vi "Create Channels From FrontPanel.vi"(8 "error in (no error)":errorcluster, 11 "Controls[]":refnum<vi>[](array[refnum])) -> (0 "error out":errorcluster, 3 "Array":refnum<class "FPGA Channel.lvclass">[](array[class]))   [LabVIEW 2014, in "FPGA Module editor node.lvclass"]
uses:
  FPGA Module editor node.lvclass
  fpga channel/FPGA Channel.lvclass
  <vilib>/NI/Tag Bus Module Framework/channel/channel classification.ctl
  <vilib>/Utility/VariantDataType/Type.ctl
  <vilib>/NI/Tag Bus/tag/Data Type.ctl
  <vilib>/NI/Tag Bus/tag/tag descriptor.lvclass/tag descriptor.ctl
  fpga channel/FPGA Channel.lvclass/FPGA Channel.ctl
  <vilib>/NI/Tag Bus Module Framework/channel/TBM channel.lvclass/TBM channel.ctl
  <vilib>/NI/Tag Bus/tag/write tag name.vi
  <vilib>/NI/Tag Bus/tag/write data type.vi
  fpga channel/Write FXP type.vi
  <vilib>/NI/Tag Bus Module Framework/channel/Write channel classification.vi
  <vilib>/NI/Tag Bus Module Framework/channel/TBM channel.lvclass
  <vilib>/Utility/VariantDataType/VariantType.lvlib
  <vilib>/NI/Tag Bus/tag/tag descriptor.lvclass
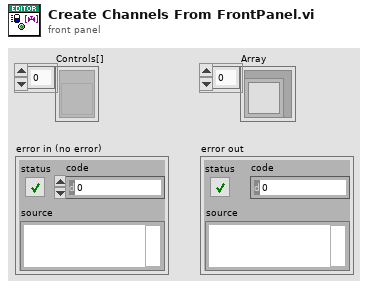
[diagram p1: front panel]
types:
  T1 = typedef "TBM channel.lvclass/channel classification.ctl" = enum16{"input data", "output data", "processing parameter", "processing result"}
  T2 = typedef "tag bus.lvlib/tag descriptor.lvclass/Data Type.ctl" = enum16{"Double", "Single", "I64", "I32", "I16", "I8", "U64", "U32", "U16", "U8", "Boolean", "String", "Array of Double", "Array of Single", "Array of I64", "Array of I32", "Array of I16", "Array of I8", "Array of U64", "Array of U32", "Array of U16", "Array of U8", "Array of Boolean", "Array of String"}
  T3 = typedef "VariantType.lvlib/Type.ctl" = enum8{"Invalid Type", "Void", "I8", "I16", "I32", "I64", "U8", "U16", "U32", "U64", "Single Float", "Double Float", "Extended Float", "Single Complex", "Double Complex", "Extended Complex", "Enum U8", "Enum U16", "Enum U32", "Enum U64", "Single Float With Unit", "Double Float With Unit", "Extended Float With Unit", "Single Complex with Unit", "Double Complex with Unit", "Extended Complex with Unit", "Boolean", "String", "Path", "Picture", "Tag", "Array", "Cluster", "Variant", "LV Variant", "Waveform", "Timestamp", "Digital Waveform", "Digital Data", "ExpressData", "Refnum", "External Data", "VI", "Poly VI", "LabVIEW Class Instance", "Fixed Point"}
  T4 = typedef "LVFixedPointRepBitsTypeDef.ctl" = cluster{"Signed":bool, "Word Length":u32, "Integer Word Length":i32}
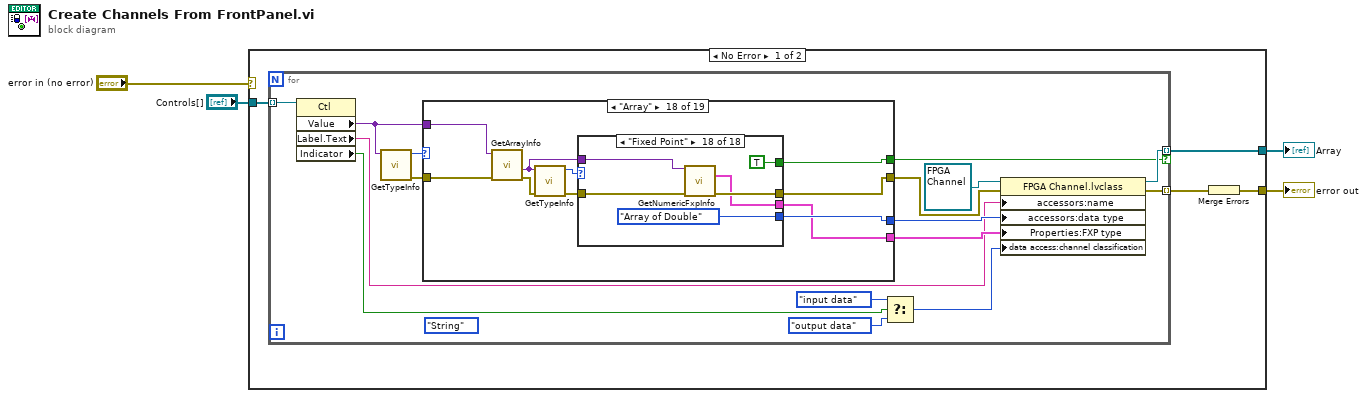
[diagram p0: block diagram]
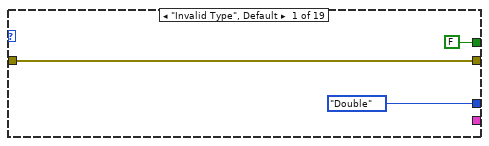
[diagram p2: hidden frame]
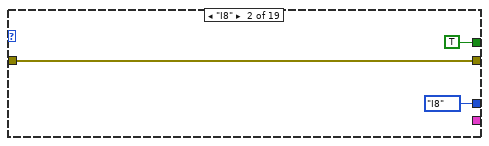
[diagram p3: hidden frame]
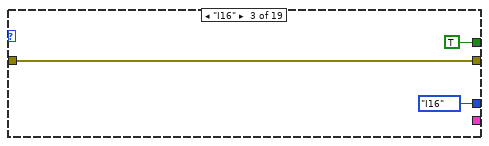
[diagram p4: hidden frame]
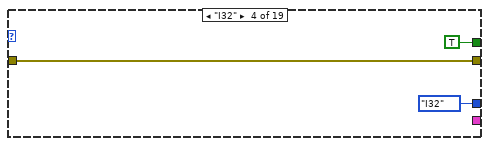
[diagram p5: hidden frame]
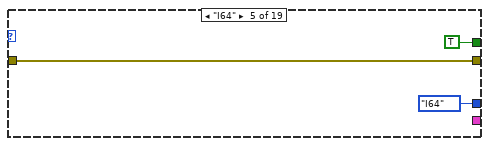
[diagram p6: hidden frame]
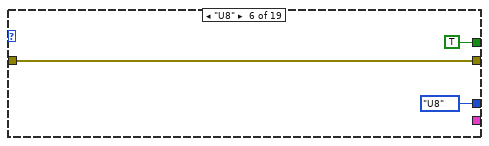
[diagram p7: hidden frame]
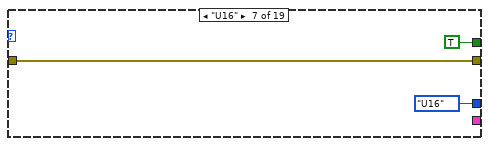
[diagram p8: hidden frame]
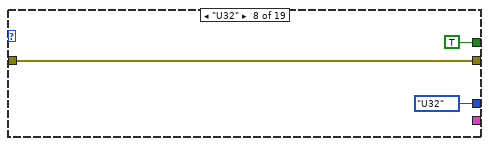
[diagram p9: hidden frame]
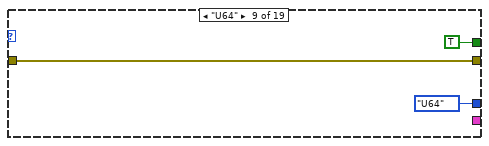
[diagram p10: hidden frame]
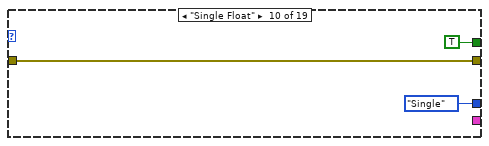
[diagram p11: hidden frame]
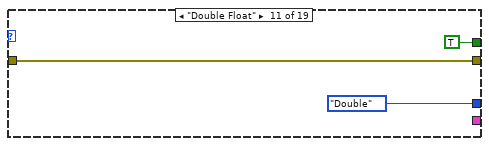
[diagram p12: hidden frame]
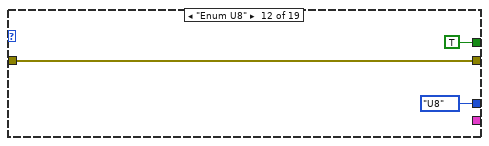
[diagram p13: hidden frame]
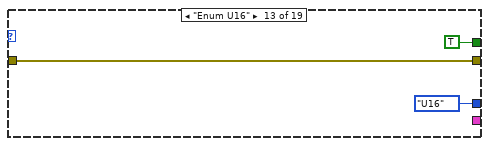
[diagram p14: hidden frame]
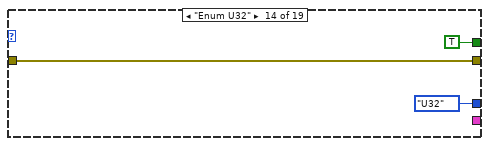
[diagram p15: hidden frame]
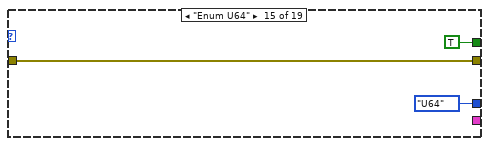
[diagram p16: hidden frame]
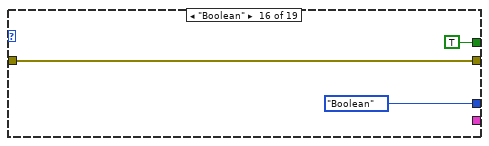
[diagram p17: hidden frame]
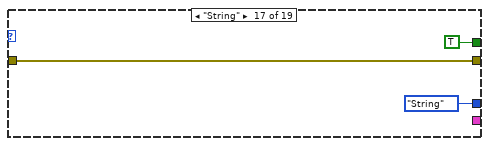
[diagram p18: hidden frame]
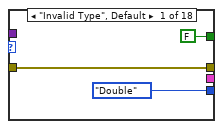
[diagram p19: hidden frame]
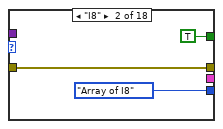
[diagram p20: hidden frame]
diagram:
  n1 = case shown="No Error" "error in (no error)" {
    selector: "error in (no error)" -> [_ w150]
    tunnel: "Controls[]" -> [w8 _]
    tunnel: [w6 w150] -> w4
    tunnel: [w5 refnum<class "FPGA Channel.lvclass">[] []] -> w3
    frame No Error {
      n2 = for {
        tunnel: w8 -> [w24] mode=indexing
        tunnel: [w19] -> w5 mode=indexing if=w18
        tunnel: [w9] -> w7 mode=indexing
        (unwired) Type."String" ("Type Enum")
        n3 = property class="Ctl"(reference=w24) -> ("Value"=w13:variant, "Label.Text"=w11:string, "Indicator"=w14:bool)  [unwired: 1 in, 2 out]
        n4 = call <vilib>:"GetTypeInfo.vi"("Variant"=w13) -> ("error out"=w20:errorcluster, "Type Enum"=w23:T3)  [unwired: 6 in, 3 out]
        n5 = case shown="\"Array\"" w23 {
          tunnel: [w27 w28 w31 w34 w37 w40 w43 w46 w49 w52 w55 w58 w61 w64 w67 w70 w73 w78 w147] -> w21
          tunnel: w20 -> [w27 w28 w31 w34 w37 w40 w43 w46 w49 w52 w55 w58 w61 w64 w67 w70 w73 w84 w148]
          tunnel: [FALSE TRUE TRUE TRUE TRUE TRUE TRUE TRUE TRUE TRUE TRUE TRUE TRUE TRUE TRUE TRUE TRUE w80 TRUE] -> w18
          tunnel: [Data_Type."Double" ("data type") Data_Type."I8" ("data type") Data_Type."I16" ("data type") Data_Type."I32" ("data type") Data_Type."I64" ("data type") Data_Type."U8" ("data type") Data_Type."U16" ("data type") Data_Type."U32" ("data type") Data_Type."U64" ("data type") Data_Type."Single" ("data type") Data_Type."Double" ("data type") Data_Type."U8" ("data type") Data_Type."U16" ("data type") Data_Type."U32" ("data type") Data_Type."U64" ("data type") Data_Type."Boolean" ("data type") Data_Type."String" ("data type") w79 Data_Type."Double" ("data type")] -> w17
          tunnel: w13 -> [_ _ _ _ _ _ _ _ _ _ _ _ _ _ _ _ _ w85 w146]
          tunnel: [_ _ _ _ _ _ _ _ _ _ _ _ _ _ _ _ _ w77 w145] -> w12
          frame "Invalid Type", Default {
          }
          frame "I8" {
          }
          frame "I16" {
          }
          frame "I32" {
          }
          frame "I64" {
          }
          frame "U8" {
          }
          frame "U16" {
          }
          frame "U32" {
          }
          frame "U64" {
          }
          frame "Single Float" {
          }
          frame "Double Float" {
          }
          frame "Enum U8" {
          }
          frame "Enum U16" {
          }
          frame "Enum U32" {
          }
          frame "Enum U64" {
          }
          frame "Boolean" {
          }
          frame "String" {
          }
          frame "Array" {
            n6 = call <vilib>:"GetArrayInfo.vi"("error in (no error)"=w84, "Variant"=w85) -> ("error out"=w83:errorcluster, "ArrayElement"=w82:variant)  [unwired: 6 in, 2 out]
            n7 = call <vilib>:"GetTypeInfo.vi"("error in (no error)"=w83, "Variant"=w82) -> ("error out"=w81:errorcluster, "Type Enum"=w76:T3)  [unwired: 5 in, 3 out]
            n8 = case shown="\"Fixed Point\"" w76 {
              tunnel: [w88 w89 w92 w95 w98 w101 w104 w107 w110 w113 w116 w119 w122 w125 w128 w131 w134 w141] -> w78
              tunnel: w81 -> [w88 w89 w92 w95 w98 w101 w104 w107 w110 w113 w116 w119 w122 w125 w128 w131 w134 w142]
              tunnel: [FALSE TRUE TRUE TRUE TRUE TRUE TRUE TRUE TRUE TRUE TRUE TRUE TRUE TRUE TRUE TRUE TRUE TRUE] -> w80
              tunnel: [Data_Type."Double" ("data type") Data_Type."Array of I8" ("data type") Data_Type."Array of I16" ("data type") Data_Type."Array of I32" ("data type") Data_Type."Array of I64" ("data type") Data_Type."Array of U8" ("data type") Data_Type."Array of U16" ("data type") Data_Type."Array of U32" ("data type") Data_Type."Array of U64" ("data type") Data_Type."Array of Single" ("data type") Data_Type."Array of Double" ("data type") Data_Type."Array of U8" ("data type") Data_Type."Array of U16" ("data type") Data_Type."Array of U32" ("data type") Data_Type."Array of U64" ("data type") Data_Type."Array of Boolean" ("data type") Data_Type."Array of String" ("data type") Data_Type."Array of Double" ("data type")] -> w79
              tunnel: w82 -> [_ _ _ _ _ _ _ _ _ _ _ _ _ _ _ _ _ w140]
              tunnel: [_ _ _ _ _ _ _ _ _ _ _ _ _ _ _ _ _ w139] -> w77
              frame "Invalid Type", Default {
              }
              frame "I8" {
              }
              frame "I16" {
              }
              frame "I32" {
              }
              frame "I64" {
              }
              frame "U8" {
              }
              frame "U16" {
              }
              frame "U32" {
              }
              frame "U64" {
              }
              frame "Single Float" {
              }
              frame "Double Float" {
              }
              frame "Enum U8" {
              }
              frame "Enum U16" {
              }
              frame "Enum U32" {
              }
              frame "Enum U64" {
              }
              frame "Boolean" {
              }
              frame "String" {
              }
              frame "Fixed Point" {
                n9 = call <vilib>:"GetNumericFxpInfo.vi"("Variant"=w140, "error in (no error)"=w142) -> ("FxpRepresentation"=w139:T4, "error out"=w141:errorcluster)  [unwired: 9 in, 3 out]
              }
            }
          }
          frame "Fixed Point" {
            n10 = call <vilib>:"GetNumericFxpInfo.vi"("Variant"=w146, "error in (no error)"=w148) -> ("FxpRepresentation"=w145:T4, "error out"=w147:errorcluster)  [unwired: 9 in, 3 out]
          }
        }
        n11 = Select(t=channel_classification."input data" ("channel classification"), s=w14, f=channel_classification."output data" ("channel classification")) -> (s? t:f=w10:T1)
        n12 = property class="FPGA Channel.lvclass"(reference=refnum<class "FPGA Channel.lvclass"> refnum ("FPGA Channel.lvclass"), error in=w21, "accessors:name"=w11, "accessors:data type"=w17, "Properties:FXP type"=w12, "data access:channel classification"=w10) -> (reference out=w19:refnum<class "FPGA Channel.lvclass">, error out=w9:errorcluster)
      }
      n13 = Merge Errors(w7) -> (w6:errorcluster)
    }
    frame Error {
    }
  }
  "error out" <- w4
  "Array" <- w3
